vi "1motorPwmTest.vi"() -> ()   [LabVIEW 2020]
uses:
  <vilib>/CISH Robotics/L4VMX TitanQuad/Motor ID.ctl
  <vilib>/CISH Robotics/L4VMX TitanQuad/TitanQuad.lvclass
panel:
  in  "Motor ID":T1
  out "Counter Value":i32
  in  "Stop Button":bool
  in  "motorSpeed (PWM) [-255~255]":dbl(slide) scale=-255.0..255.0
  # "M0-M2 「左、右、後輪」 正轉逆時針\nM3 正轉爪向上"
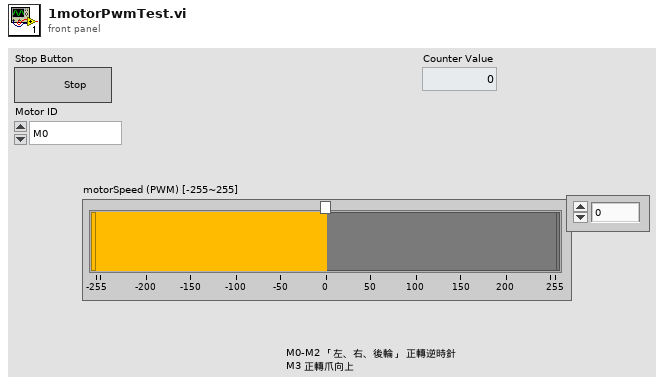
[diagram p1: front panel]
types:
  T1 = typedef "TitanQuad.lvlib/TitanQuad.lvclass/Motor ID.ctl" = enum16{"M0", "M1", "M2", "M3"}
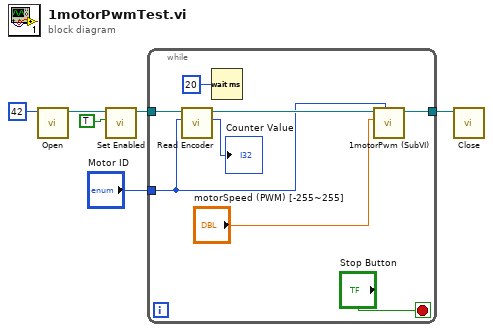
[diagram p0: block diagram]
diagram:
  n1 = call <vilib>:"Open.vi"("Titan ID (42)"=u8 42) -> ("TitanQuad Object"=w6:refnum<class "TitanQuad.lvclass">)  [unwired: 9 in, 1 out]
  n2 = call <vilib>:"Set Enabled.vi"("Enable"=TRUE, "TitanQuad Object"=w6) -> ("TitanQuad Object"=w5:refnum<class "TitanQuad.lvclass">)  [unwired: 8 in, 1 out]
  n3 = while {
    tunnel: w5 -> [w10]
    tunnel: [w14] -> w4
    tunnel: "Motor ID" -> [w7]
    stop <- "Stop Button" stop-if-true
    n4 = call <vilib>:"Read Encoder.vi"("Motor ID"=w7, "TitanQuad Object"=w10) -> ("Counter Value"=→"Counter Value":i32, "TitanQuad Object"=w9:refnum<class "TitanQuad.lvclass">)  [unwired: 7 in, 1 out]
    n5 = Wait (ms)(milliseconds to wait=u32 20) -> ()  [unwired: 1 out]
    n6 = call "1motorPwm (SubVI).vi"("Motor ID"=w7, "motorPwmSpeed"="motorSpeed (PWM) [-255~255]", "TitanQuad in"=w9) -> ("TitanQuad out"=w14:refnum<class "TitanQuad.lvclass">)  [unwired: 7 in, 1 out]
  }
  n7 = call <vilib>:"Close.vi"("TitanQuad Object"=w4) -> ()  [unwired: 10 in, 1 out]
